vi "CAPTH-Save History.vi"(0 "Params":T5={"Stimulus"={"EAR"=enum."RIGHT", "HI FREQ"=0.0, "LO FREQ"=0.0, "FREQ STEP"=0, "Rep Rate (/s)"=0.0, "Alternate Polarity"=FALSE, "# CYCLES"=0, "Duration (ms)"=0.0, "Ramp (ms)"=0.0}, "Response"={"Averages (3dB steps)"=0, "Time Window (ms)"=0.0, "dt (us)"=0.0, "Grass gain"=0.0, "CRITERION (mV)"=0.0, "CEILING (dB atten)"=0.0, "Use previous"=FALSE, "Save avgs"=FALSE, "Save raw"=FALSE, "Save history"=FALSE, "CEILING (dB SPL)"=6.0}} {"Response"."CRITERION (mV)" format="%.2f"; "Response"."Time Window (ms)" format="%.2f"}, 5 "State":T2) -> (15 "error out":errorcluster)   [LabVIEW 2020]
uses:
  Typedefs/CAPTH-Parameters.ctl
  Typedefs/CAPTH-Stimulus.ctl
  Typedefs/CAPTH-Response.ctl
  Typedefs/CAPTH-Analysis State.ctl
  Typedefs/CAPTH-History.ctl
  Typedefs/CAPTH-StimCon.ctl
panel:
  in  "CAPTH":T1
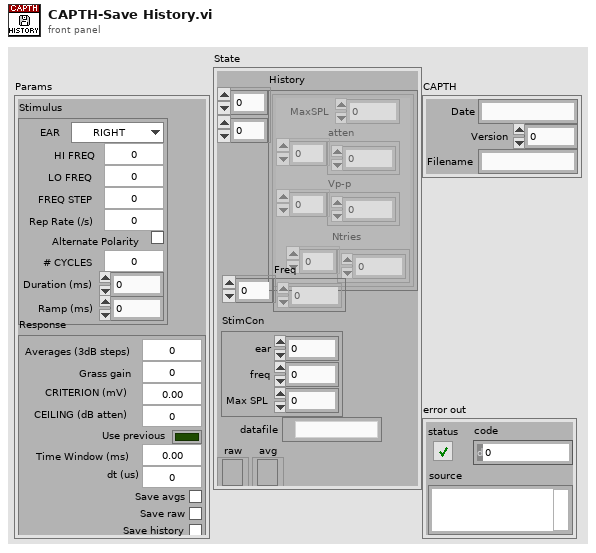
[diagram p1: front panel]
types:
  T1 = cluster{"Date":string, "Version":i32, "Filename":string}
  T2 = typedef "CAPTH-Analysis State.ctl" = cluster{"History":T3, "Freq":dbl[], "StimCon":T4, "datafile":path, "raw":refnum<file>, "avg":refnum<file>}
  T3 = typedef "CAPTH-History.ctl" = cluster{"MaxSPL":dbl, "atten":dbl[], "Vp-p":dbl[], "Ntries":i32[]}[][]
  T4 = typedef "CAPTH-StimCon.ctl" = cluster{"ear":i32, "freq":i32, "Max SPL":dbl}
  T5 = typedef "CAPTH-Parameters.ctl" = cluster{"Stimulus":T6, "Response":T7}
  T6 = typedef "CAPTH-Stimulus.ctl" = cluster{"EAR":enum16{"RIGHT", "LEFT\n", "ALTERNATE"}, "HI FREQ":dbl, "LO FREQ":dbl, "FREQ STEP":u8, "Rep Rate (/s)":dbl, "Alternate Polarity":bool, "# CYCLES":u8, "Duration (ms)":dbl, "Ramp (ms)":dbl}
  T7 = typedef "CAPTH-Response.ctl" = cluster{"Averages (3dB steps)":i32, "Time Window (ms)":dbl, "dt (us)":dbl, "Grass gain":dbl, "CRITERION (mV)":dbl, "CEILING (dB atten)":dbl, "Use previous":bool, "Save avgs":bool, "Save raw":bool, "Save history":bool, "CEILING (dB SPL)":dbl}
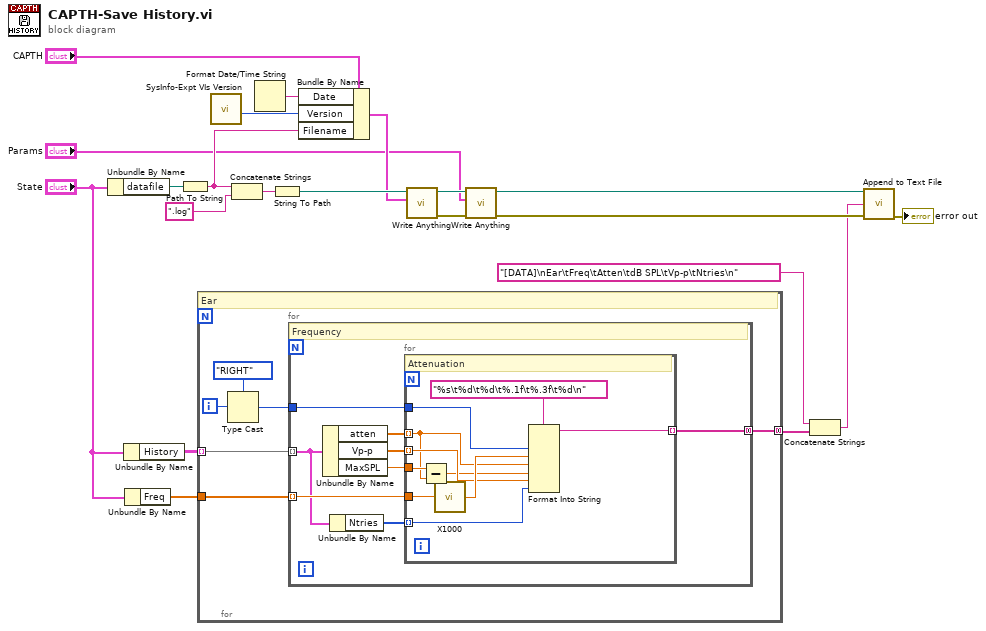
[diagram p0: block diagram]
diagram:
  n1 = Unbundle By Name("State") -> ("datafile"=w18:path)
  n2 = Unbundle By Name("State") -> ("History"=w6:T3)
  n3 = Unbundle By Name("State") -> ("Freq"=w4:dbl[])
  n4 = Path To String(path=w18) -> (string=w17:string)
  n5 = for {
    tunnel: w6 -> [w27] mode=indexing
    tunnel: w4 -> [w23]
    tunnel: [w22] -> w3 mode=concatenating
    i -> [w26]
    # "Ear"
    n6 = Type Cast(type=enum16{"RIGHT", "LEFT\n", "ALTERNATE"}."RIGHT" ("Stimulus.EAR"), x=w26) -> (*(type *) &x=w24:enum16{"RIGHT", "LEFT\n", "ALTERNATE"})
    n7 = for {
      tunnel: w27 -> [w29] mode=indexing
      tunnel: w23 -> [w31] mode=indexing
      tunnel: w24 -> [w32]
      tunnel: [w30] -> w22 mode=concatenating
      # "Frequency"
      n8 = Unbundle By Name(w29) -> ("atten"=w35:dbl[], "Vp-p"=w34:dbl[], "MaxSPL"=w33:dbl)
      n9 = Unbundle By Name(w29) -> ("Ntries"=w28:i32[])
      n10 = for {
        tunnel: w35 -> [w39] mode=indexing
        tunnel: w34 -> [w41] mode=indexing
        tunnel: w33 -> [w40]
        tunnel: w32 -> [w44]
        tunnel: w31 -> [w43]
        tunnel: [w37] -> w30 mode=indexing
        tunnel: w28 -> [w36] mode=indexing
        # "Attenuation"
        n11 = Subtract(x=w40, y=w39) -> (x-y=w38:dbl)
        n12 = call "X1000.vi"("X"=w43) -> ("X/1000"=w42:dbl)
        n13 = Format Into String(format string="%s\t%d\t%d\t%.1f\t%.3f\t%d\n", w44, w42, w39, w38, w41, w36) -> (resulting string=w37:string)  [unwired: 2 in, 1 out]
      }
    }
  }
  n14 = call "SysInfo-Expt VIs Version.vi"() -> ("Expt VIs Version out"=w20:i32)  [unwired: 11 in]
  n15 = Concatenate Strings(w17, ".log" ("string")) -> (w15:string)
  n16 = Format Date/Time String() -> (date/time string=w21:string)  [unwired: 3 in]
  n17 = String To Path(string=w15) -> (path=w14:path)
  n18 = Bundle By Name(cluster="CAPTH", "Date"=w21, "Version"=w20, "Filename"=w17) -> (w13:T1)
  n19 = call "Write Anything.vi"("Anything"=w13, "Path (dialog)"=w14) -> ("Error Out"=w12:errorcluster, "Path out"=w11:path)  [unwired: 8 in]
  n20 = call "Write Anything.vi"("Error In"=w12, "Anything"="Params", "Path (dialog)"=w11) -> ("Error Out"=w8:errorcluster, "Path out"=w9:path)  [unwired: 7 in]
  n21 = Concatenate Strings("[DATA]\nEar\tFreq\tAtten\tdB SPL\tVp-p\tNtries\n", w3) -> (w1:string)
  n22 = call "Append to Text File.vi"("file path"=w9, "text"=w1, "error in (no error)"=w8) -> ("error out"=→"error out":errorcluster)  [unwired: 11 in, 1 out]
